vi "creaRefTimerG3.vi"(8 "error in (no error)":errorcluster) -> (0 "error out":errorcluster)   [LabVIEW 2018]
uses:
  Global/TimerReferences.vi
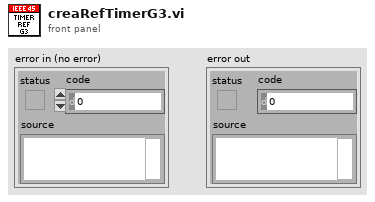
[diagram p1: front panel]
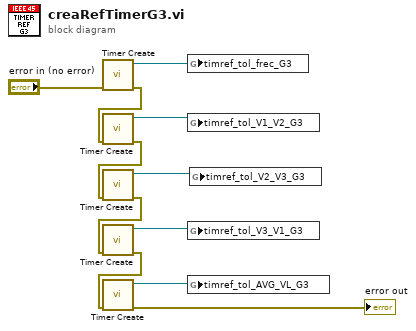
[diagram p0: block diagram]
diagram:
  n1 = call "Timer Create.vi"("error in (no error)"="error in (no error)") -> ("error out"=w6:errorcluster, "Timer reference out"=w11:refnum<data-value>)  [unwired: 9 in]
  n2 = call "Timer Create.vi"("error in (no error)"=w6) -> ("error out"=w5:errorcluster, "Timer reference out"=w10:refnum<data-value>)  [unwired: 9 in]
  n3 = call "Timer Create.vi"("error in (no error)"=w5) -> ("error out"=w4:errorcluster, "Timer reference out"=w9:refnum<data-value>)  [unwired: 9 in]
  n4 = call "Timer Create.vi"("error in (no error)"=w4) -> ("error out"=w3:errorcluster, "Timer reference out"=w8:refnum<data-value>)  [unwired: 9 in]
  n5 = call "Timer Create.vi"("error in (no error)"=w3) -> ("error out"=→"error out":errorcluster, "Timer reference out"=w7:refnum<data-value>)  [unwired: 9 in]
  n6 = global write "TimerReferences.vi" "timref_tol_frec_G3"(w11) -> ()
  n7 = global write "TimerReferences.vi" "timref_tol_V1_V2_G3"(w10) -> ()
  n8 = global write "TimerReferences.vi" "timref_tol_V3_V1_G3"(w8) -> ()
  n9 = global write "TimerReferences.vi" "timref_tol_AVG_VL_G3"(w7) -> ()
  n10 = global write "TimerReferences.vi" "timref_tol_V2_V3_G3"(w9) -> ()
